vi "Set Address.vi"(10 "Column":i32, 11 "Row":i32) -> (3 "2D Array Index":refnum<class "2D Array.lvclass">)   [LabVIEW 2019, in "2D Array.lvclass"]
uses:
  2D Array.lvclass
  2D Array.lvclass/2D Array.ctl
  Write Row.vi
  Write Column.vi
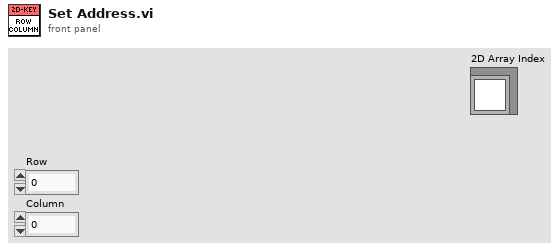
[diagram p1: front panel]
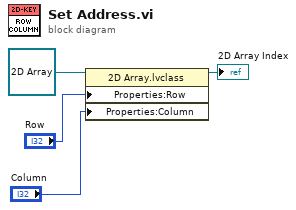
[diagram p0: block diagram]
diagram:
  n1 = property class="2D Array.lvclass"(reference=refnum<class "2D Array.lvclass"> refnum ("2D Array.lvclass"), "Properties:Row"="Row", "Properties:Column"="Column") -> (reference out=→"2D Array Index":refnum<class "2D Array.lvclass">)  [unwired: 1 in, 1 out]
